vi "Stop.vi"(8 "error in (no error)":errorcluster, 11 "VISA GPS in":refnum<class "VISA GPS.lvclass">) -> (0 "error out":errorcluster, 3 "VISA GPS out":refnum<class "VISA GPS.lvclass">)   [LabVIEW 2020, in "nmea.lvlib" / "VISA GPS.lvclass"]
uses:
  VISA GPS.lvclass
  VISA GPS.lvclass/VISA GPS.ctl
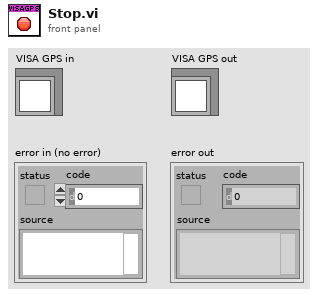
[diagram p1: front panel]
types:
  T1 = typedef "nmea.lvlib/VISA GPS.lvclass/Ref Data.ctl" = cluster{"Close":bool}
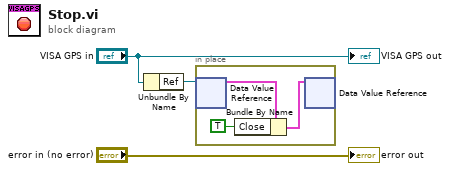
[diagram p0: block diagram]
diagram:
  n1 = Unbundle By Name("VISA GPS in") -> ("Ref"=w2:refnum<data-value>)
  n2 = in-place {
    n3 = in-place-dvr #1(w2) -> (w6:T1)  [unwired: 1 out]
    n4 = Bundle By Name(cluster=w6, "Close"=TRUE) -> (w5:T1)
    n5 = in-place-dvr #1(w5) -> ()  [unwired: 2 out]
  }
  "error out" <- "error in (no error)"
  "VISA GPS out" <- "VISA GPS in"
